vi "subtable to data table.vi"(11 "subtable":T1) -> (3 "full data table":T2)   [LabVIEW 2013, in "Tag Bus Web Interface configuration.lvclass"]
uses:
  Tag Bus Web Interface configuration.lvclass
  <vilib>/NI/Tag Bus/table/data table.ctl
  subtable.ctl
  <vilib>/NI/Tag Bus/table/data table.lvlib
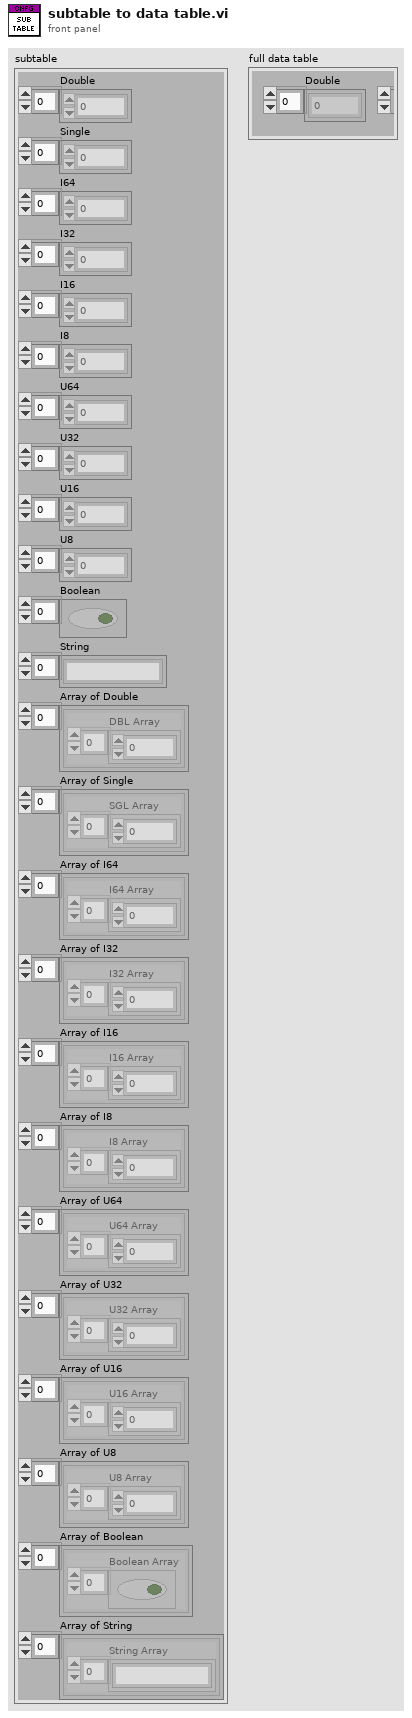
[diagram p1: front panel]
types:
  T1 = typedef "Tag Bus Web Interface configuration.lvclass/subtable.ctl" = cluster{"Double":dbl[], "Single":sgl[], "I64":i64[], "I32":i32[], "I16":i16[], "I8":i8[], "U64":u64[], "U32":u32[], "U16":u16[], "U8":u8[], "Boolean":bool[], "String":string[], "Array of Double":cluster{"DBL Array":dbl[]}[], "Array of Single":cluster{"SGL Array":sgl[]}[], "Array of I64":cluster{"I64 Array":i64[]}[], "Array of I32":cluster{"I32 Array":i32[]}[], "Array of I16":cluster{"I16 Array":i16[]}[], "Array of I8":cluster{"I8 Array":i8[]}[], "Array of U64":cluster{"U64 Array":u64[]}[], "Array of U32":cluster{"U32 Array":u32[]}[], "Array of U16":cluster{"U16 Array":u16[]}[], "Array of U8":cluster{"U8 Array":u8[]}[], "Array of Boolean":cluster{"Boolean Array":bool[]}[], "Array of String":cluster{"String Array":string[]}[]}
  T2 = typedef "tag bus.lvlib/data table.lvlib/data table.ctl" = cluster{"Double":dbl[], "Single":sgl[], "I64":i64[], "I32":i32[], "I16":i16[], "I8":i8[], "U64":u64[], "U32":u32[], "U16":u16[], "U8":u8[], "Boolean":bool[], "String":string[], "Array of Double":cluster{"DBL Array":dbl[]}[], "Array of Single":cluster{"SGL Array":sgl[]}[], "Array of I64":cluster{"I64 Array":i64[]}[], "Array of I32":cluster{"I32 Array":i32[]}[], "Array of I16":cluster{"I16 Array":i16[]}[], "Array of I8":cluster{"I8 Array":i8[]}[], "Array of U64":cluster{"U64 Array":u64[]}[], "Array of U32":cluster{"U32 Array":u32[]}[], "Array of U16":cluster{"U16 Array":u16[]}[], "Array of U8":cluster{"U8 Array":u8[]}[], "Array of Boolean":cluster{"Boolean Array":bool[]}[], "Array of String":cluster{"String Array":string[]}[]}
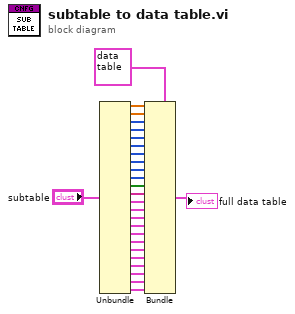
[diagram p0: block diagram]
diagram:
  n1 = Unbundle("subtable") -> ("Double"=w27:dbl[], "Single"=w26:sgl[], "I64"=w25:i64[], "I32"=w24:i32[], "I16"=w23:i16[], "I8"=w22:i8[], "U64"=w21:u64[], "U32"=w20:u32[], "U16"=w19:u16[], "U8"=w18:u8[], "Boolean"=w17:bool[], "String"=w16:string[], "Array of Double"=w15:cluster{"DBL Array":dbl[]}[], "Array of Single"=w14:cluster{"SGL Array":sgl[]}[], "Array of I64"=w13:cluster{"I64 Array":i64[]}[], "Array of I32"=w12:cluster{"I32 Array":i32[]}[], "Array of I16"=w11:cluster{"I16 Array":i16[]}[], "Array of I8"=w10:cluster{"I8 Array":i8[]}[], "Array of U64"=w9:cluster{"U64 Array":u64[]}[], "Array of U32"=w8:cluster{"U32 Array":u32[]}[], "Array of U16"=w7:cluster{"U16 Array":u16[]}[], "Array of U8"=w4:cluster{"U8 Array":u8[]}[], "Array of Boolean"=w6:cluster{"Boolean Array":bool[]}[], "Array of String"=w5:cluster{"String Array":string[]}[])
  n2 = Bundle(cluster=T2 {"Double"=[], "Single"=[], "I64"=[], "I32"=[], "I16"=[], "I8"=[], "U64"=[], "U32"=[], "U16"=[], "U8"=[], "Boolean"=[], "String"=[], "Array of Double"=[], "Array of Single"=[], "Array of I64"=[], "Array of I32"=[], "Array of I16"=[], "Array of I8"=[], "Array of U64"=[], "Array of U32"=[], "Array of U16"=[], "Array of U8"=[], "Array of Boolean"=[], "Array of String"=[]} ("full data table"), "Double"=w27, "Single"=w26, "I64"=w25, "I32"=w24, "I16"=w23, "I8"=w22, "U64"=w21, "U32"=w20, "U16"=w19, "U8"=w18, "Boolean"=w17, "String"=w16, "Array of Double"=w15, "Array of Single"=w14, "Array of I64"=w13, "Array of I32"=w12, "Array of I16"=w11, "Array of I8"=w10, "Array of U64"=w9, "Array of U32"=w8, "Array of U16"=w7, "Array of U8"=w4, "Array of Boolean"=w6, "Array of String"=w5) -> (→"full data table":T2)
